vi "WPI_DMAPause.vi"(8 "error in (no error)":errorcluster, 11 "DMARef":T1) -> (0 "error out":errorcluster, 3 "DMARef":T1)   [LabVIEW 2017]
doc: "Causes the hardware to ignore the sample source in the DMA stream. Call the Start VI to unpause the stream and reinitiate the data transfer.\n\nThis software is licensed. Open the labview\\readme\\WPI Robotics Library Open Source License.txt file for more information."
uses:
  <vilib>/Rock Robotics/WPI/DMA/WPI_DMARef.ctl
  <vilib>/Rock Robotics/SystemInterfaces/DMA/FPGA_DMAWriteConfigOperation.ctl
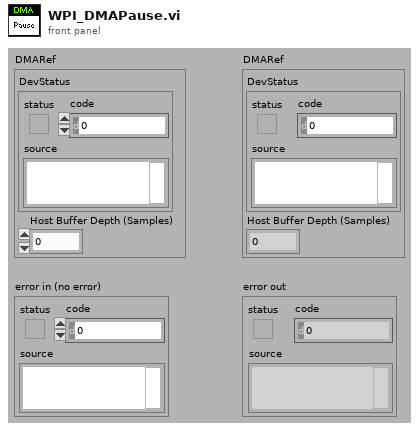
[diagram p1: front panel]
types:
  T1 = typedef "WPI_DMARef.ctl" = cluster{"DevStatus":errorcluster, "Host Buffer Depth (Samples)":u32}
  T2 = typedef "FPGA_DMAWriteConfigOperation.ctl" = enum16{"Update Pause", "Update Enable", "Update SampleClock"}
  T3 = typedef "FPGA_DMADevRef.ctl" = cluster{"DevStatus":errorcluster}
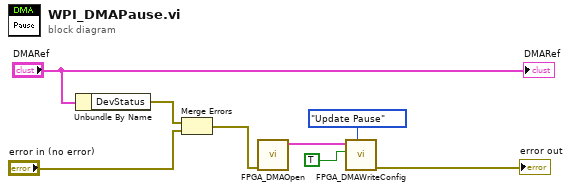
[diagram p0: block diagram]
diagram:
  n1 = Unbundle By Name("DMARef") -> ("DevStatus"=w3:errorcluster)
  n2 = Merge Errors(w3, "error in (no error)") -> (w2:errorcluster)
  n3 = call <vilib>:"FPGA_DMAOpen.vi"("error in (no error)"=w2) -> ("DMADevRef"=w5:T3)  [unwired: 10 out]
  n4 = call <vilib>:"FPGA_DMAWriteConfig.vi"("Operation"=FPGA_DMAWriteConfigOperation."Update Pause", "Pause"=TRUE, "DMADevRef"=w5) -> ("error out"=→"error out":errorcluster)  [unwired: 3 in, 5 out]
  "DMARef" <- "DMARef"
